vi "军蚁-禁用菜单功能.vi"(8 "error in":errorcluster caption="error out", 11 "菜单引用":refnum<k9>) -> (0 "error Out":errorcluster caption="error in")   [LabVIEW 2017]
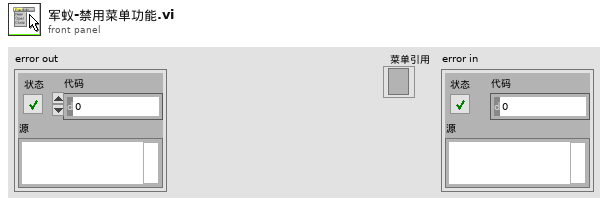
[diagram p1: front panel]
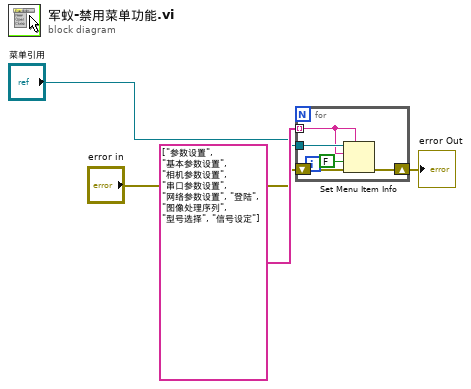
[diagram p0: block diagram]
diagram:
  n1 = for {
    tunnel: "菜单引用" -> [w9]
    tunnel: string[] ["参数设置", "基本参数设置", "相机参数设置", "串口参数设置", "网络参数设置", "登陆", "图像处理序列", "型号选择", "信号设定"] -> [w7] mode=indexing
    shift-right: [w5] -> w1
    shift-left: "error in" -> [w6]
    n2 = Set Menu Item Info(7:w7, 8:w6, 9:FALSE ("已启用"), 10:w7, 11:w9) -> (0:w5:errorcluster)  [unwired: 2 in, 1 out]
  }
  "error Out" <- w1
